vi "IR AOM word to freq - vec.vi"(1 "Frequency Word In (double vec)":u64[](array[numeric])) -> (0 "Frequency Out":dbl[](array[numeric]))   [LabVIEW 2014]
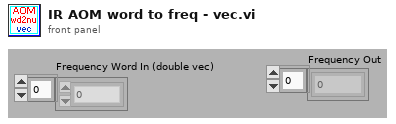
[diagram p1: front panel]
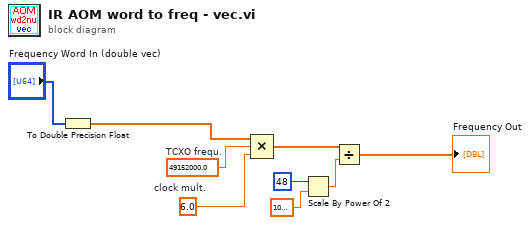
[diagram p0: block diagram]
diagram:
  w4 = 6.0  # clock mult.
  w5 = 49152000.0  # TCXO frequ.
  n1 = To Double Precision Float(number="Frequency Word In (double vec)") -> (double precision float=w7:dbl[])
  n2 = Compound Arithmetic op=MULTIPLY(w7, w5, w4) -> (w3:dbl[])
  n3 = Scale By Power Of 2(n=48, x=1000000.0 ("y")) -> (x*2^n=w1:dbl)
  n4 = Divide(x=w3, y=w1) -> (x/y=→"Frequency Out":dbl[])
